vi "VI SysLog History.vi"() -> ()   [LabVIEW 2020, in "SysLog.lvlib"]
uses:
  SysLog.lvlib
  Stoerungen/Stoermelde Tabelle.ctl
  Visualisierungs Elemente/Button.ctl
  Visualisierungs Elemente/Auswahlfeld.ctl
  SysLogSort.ctl
  Passwortverwaltung/FGV Passwort Aktion.ctl
  <vilib>/Utility/miscctls.llb/LVRowAndColumnUnsignedTypeDef.ctl
  Allgemein/allgemeine Sub-VIs.lvlib
  Sprachverwaltung/Sprachverwaltung.lvlib
  Passwortverwaltung/Passwort.lvlib
  Stoerungen/Stoerungen.lvlib
panel:
  in  "SuchString":string caption="Suche"
  in  "interne":T1 items=["alle", "nur benutzerrelevante", "nur interne"]
  out "Fehler (out)":errorcluster caption="Fehlerkonstante"
  in  "cRIO History Laden":T2
  in  "PC History Laden":T2
  in  "Richtung":T1 items=["v", "^"]
  in  "Sortierung":T1 items=["Zeit", "Code", "Typ"]
  in  "Typ":T1 items=["*", "Err+Warn", "Err", "Warn", "OK"]
  in  "Ebene":T1 items=["PC+cRIO", "PC", "cRIO"]
  in  "refresh":T2 caption="quittieren"
  out "Tabelle":T3
  # "System Log History"
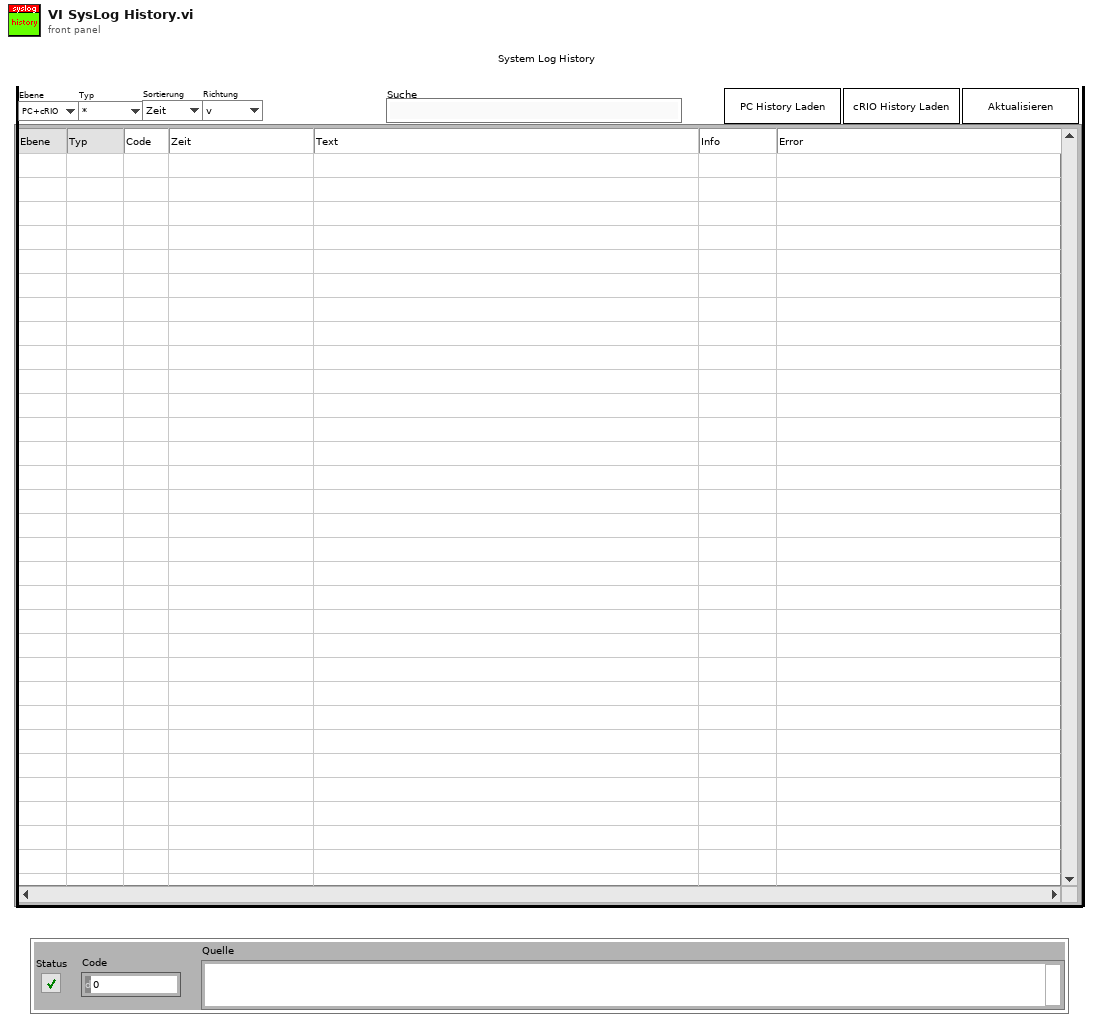
[diagram p1: front panel]
types:
  T1 = typedef "Auswahlfeld.ctl" = u16
  T2 = typedef "Button.ctl" = bool
  T3 = typedef "Stoerungen.lvlib/Stoermelde Tabelle.ctl" = string[][]
  T4 = typedef "Passwort.lvlib/FGV Passwort Aktion.ctl" = enum16{"prüfen", "setzen", "Initialisieren", "PW speichern", "lesen", "PW Änderung"}
  T5 = typedef "SysLog.lvlib/SysLogSort.ctl" = cluster{"interne":enum16{"alle", "nur benutzerrelevante", "nur interne"}, "Typ":enum16{"*", "Err+Warn", "Err", "Warn", "OK"}, "Sortierung":enum16{"Zeit", "Code", "Typ"}, "Richtung":enum16{"v", "^"}, "Filter":string}
  T6 = enum8{"Enabled", "Disabled", "Disabled and Grayed Out"}
  T7 = enum16{"alle", "nur benutzerrelevante", "nur interne"}
  T8 = typedef "LVRowAndColumnUnsignedTypeDef.ctl" = cluster{"Row":u32, "Column":u32}
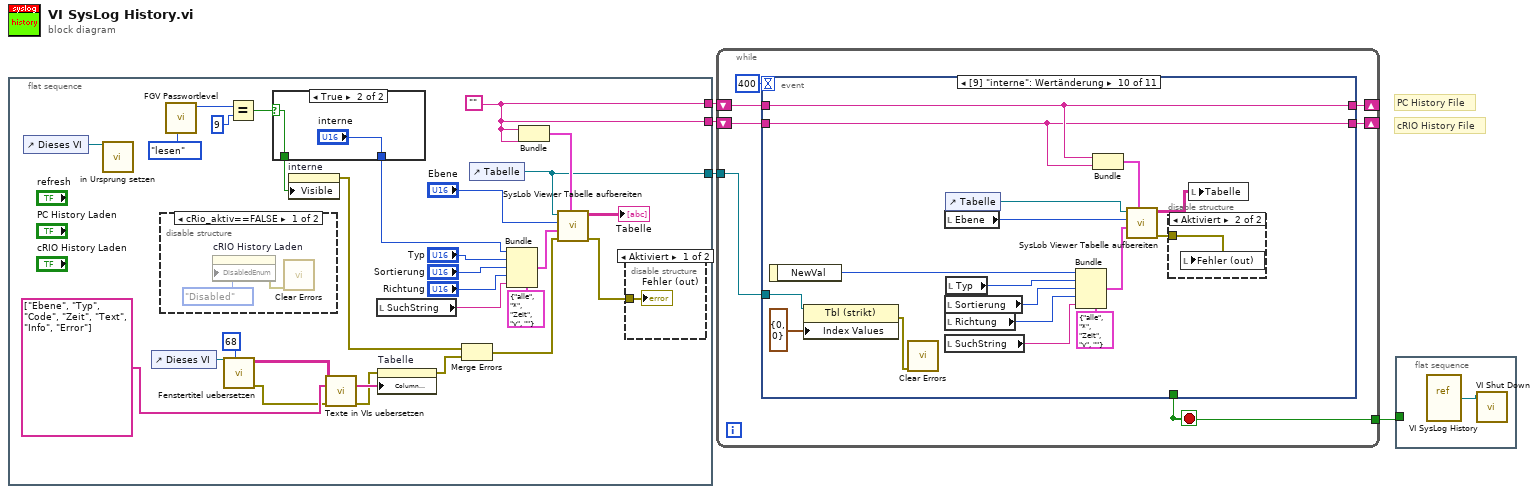
[diagram p0: block diagram]
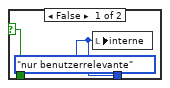
[diagram p2: hidden frame]
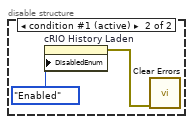
[diagram p3: hidden frame]
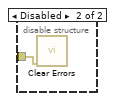
[diagram p4: hidden frame]
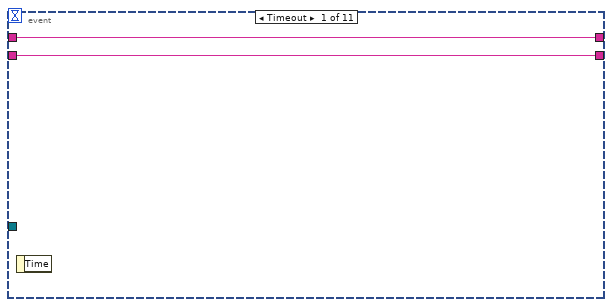
[diagram p5: hidden frame]
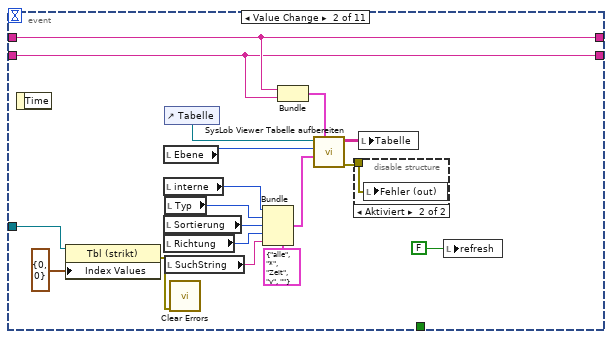
[diagram p6: hidden frame]
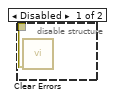
[diagram p7: hidden frame]
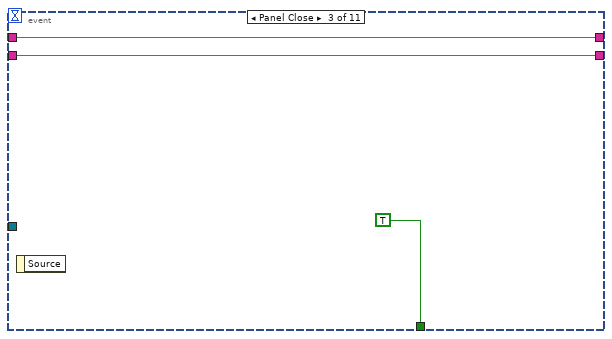
[diagram p8: hidden frame]
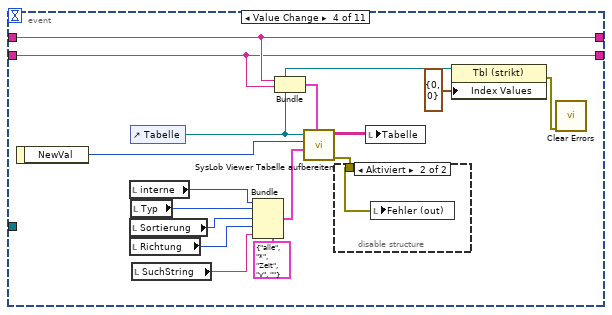
[diagram p9: hidden frame]
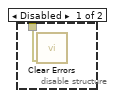
[diagram p10: hidden frame]
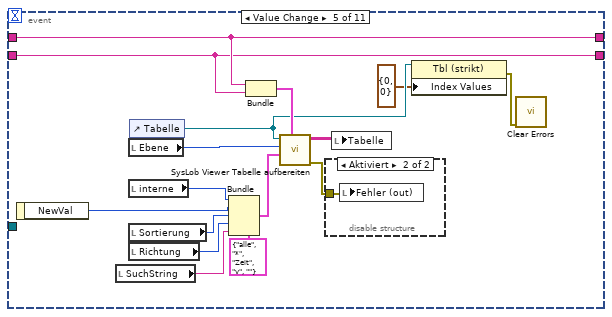
[diagram p11: hidden frame]
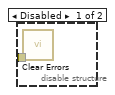
[diagram p12: hidden frame]
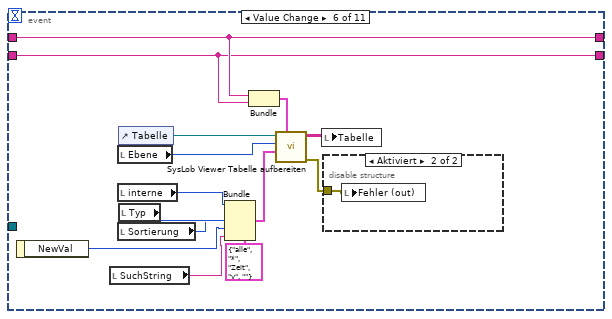
[diagram p13: hidden frame]
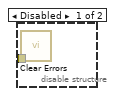
[diagram p14: hidden frame]
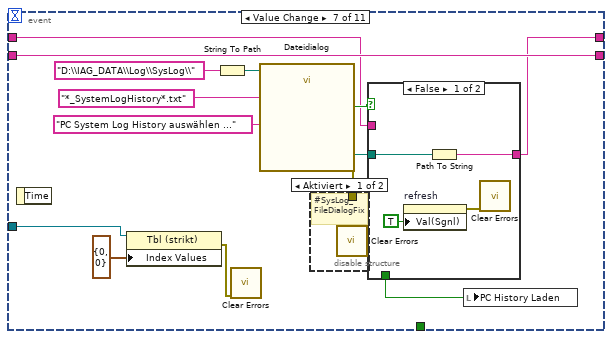
[diagram p15: hidden frame]
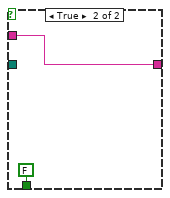
[diagram p17: hidden frame]
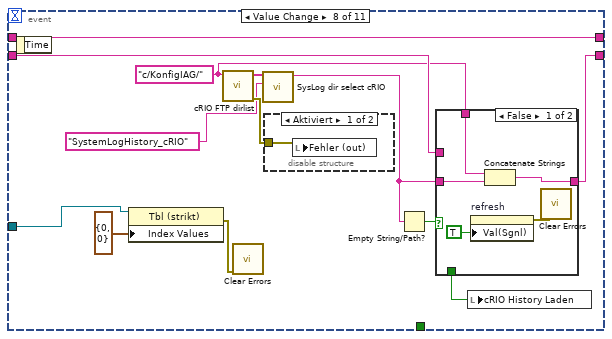
[diagram p18: hidden frame]
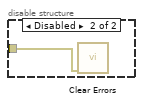
[diagram p19: hidden frame]
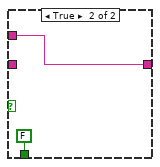
[diagram p20: hidden frame]
diagram:
  # "cRIO History File"
  # "PC History File"
  n1 = flat-sequence {
    tunnel: [w22] -> w3
    tunnel: [w22] -> w2
    tunnel: [w5] -> w1
    frame #0 {
      w22 = ""
      n2 = control-ref of="Dieses VI"() -> (w33:refnum<vi>)
      n3 = call "in Ursprung setzen.vi"("VI Referenz"=w33) -> ()  [unwired: 10 in, 1 out]
      n4 = control-ref of="Dieses VI"() -> (w16:refnum<vi>)
      n5 = disable-structure shown="cRio_aktiv==FALSE" {
        frame condition #0 {
          n6 = property on="cRIO History Laden" class="Bool. (strikt)"("DisabledEnum"=T6."Disabled" ("Deaktiviert")) -> (error out=w38:errorcluster)  [unwired: 2 in, 1 out]
          n7 = call <vilib>:"Clear Errors.vi"("error in (no error)"=w38) -> ()  [unwired: 5 in, 2 out]
        }
        frame condition #1 (active) {
          n8 = property on="cRIO History Laden" class="Bool. (strikt)"("DisabledEnum"=T6."Enabled" ("Deaktiviert")) -> (error out=w40:errorcluster)  [unwired: 2 in, 1 out]
          n9 = call <vilib>:"Clear Errors.vi"("error in (no error)"=w40) -> ()  [unwired: 5 in, 2 out]
        }
      }
      n10 = call "FGV Passwortlevel.vi"("FGV Passwort Aktion"=FGV_Passwort_Aktion."lesen") -> ("aktueller Level"=w19:i16)  [unwired: 3 in, 7 out]
      n11 = call "Fenstertitel uebersetzen.vi"("Index (Seite)"=68, "Dieses VI"=w16) -> ("error out"=w8:errorcluster, "Sprachliste"=w9:string[][])  [unwired: 6 in, 2 out]
      n12 = Equal?(x=w19, y=i16 9) -> (x = y?=w17:bool)
      n13 = case shown="True" w17 {
        selector: w17 -> [w35 w37]
        tunnel: [w35 w37] -> w11
        tunnel: [w34 "interne"] -> w10
        frame False {
          w34 = T7."nur benutzerrelevante" ("interne")
          n14 = local write "interne"(w34) -> ()
        }
        frame True {
        }
      }
      n15 = property on="interne" class="Ring (strikt)"("Visible"=w11) -> (error out=w12:errorcluster)  [unwired: 2 in, 1 out]
      n16 = call "Texte in VIs uebersetzen.vi"("Sprachliste"=w9, "String-Array zum Übersetzen"=string[] ["Ebene", "Typ", "Code", "Zeit", "Text", "Info", "Error"] ("Spaltentitel[]"), "error in (no error)"=w8) -> ("String-Array zum Übersetzen"=w31:string[], "error out"=w7:errorcluster)  [unwired: 8 in, 3 out]
      n17 = local read "SuchString"() -> (w6:string)
      n18 = property on="Tabelle" class="Tbl (strikt)"(error in=w7, "Column Headers[]"=w31) -> (error out=w14:errorcluster)  [unwired: 1 in, 1 out]
      n19 = Merge Errors(w12, w14) -> (w13:errorcluster)
      n20 = control-ref of="Tabelle"() -> (w5:refnum<vi>)
      n21 = Bundle(cluster=T5 {"interne"=enum."alle", "Typ"=enum."*", "Sortierung"=enum."Zeit", "Richtung"=enum."v", "Filter"=""} ("Cluster (in)"), "interne"=w10, "Typ"="Typ", "Sortierung"="Sortierung", "Richtung"="Richtung", "Filter"=w6) -> (w30:T5)
      n22 = Bundle(w22, w22) -> (w21:cluster{string, string})  [unwired: 1 in]
      n23 = call "SysLob Viewer Tabelle aufbereiten.vi"("Cluster PC cRIO History File"=w21, "Fehler (in)"=w13, "Cluster (in)"=w30, "Ebene"="Ebene", "Table (Eingang)"=w5) -> ("Fehler (out)"=w23:errorcluster, "Array-Typ (2D Dbl) out"=→"Tabelle":string[][])  [unwired: 5 in]
      n24 = disable-structure shown="Aktiviert" {
        disable-tunnel: w23 -> [w42 w43]
        frame Enabled {
          "Fehler (out)" <- w42
        }
        frame Disabled {
          n25 = call <vilib>:"Clear Errors.vi"("error in (no error)"=w43) -> ()  [unwired: 5 in, 2 out]
        }
      }
    }
  }
  n26 = while {
    tunnel: [w49] -> w4
    shift-right: [w47] -> _
    shift-left: w3 -> [w48]
    shift-right: [w45] -> _
    shift-left: w2 -> [w46]
    tunnel: w1 -> [w44]
    stop <- w49 stop-if-true
    n27 = event shown="[9] \"interne\": Wertänderung" {
      selector: _ -> [_ _ _ _ _ _ _ _ _ _ _]
      dyn-events: _ -> [_ _ _ _ _ _ _ _ _ _ _]
      timeout: 400 -> [_ _ _ _ _ _ _ _ _ _ _]
      tunnel: [_ _ TRUE _ _ _ _ _ _ _ _] -> w49
      tunnel: w48 -> [w52 w61 w74 w84 w101 w116 w134 w161 w175 w201 w219]
      tunnel: [w52 w61 w74 w84 w101 w116 w133 w161 w175 w201 w219] -> w47
      tunnel: w46 -> [w51 w60 w73 w83 w100 w115 w141 w160 w174 w200 w218]
      tunnel: [w51 w60 w73 w83 w100 w115 w141 w159 w174 w200 w218] -> w45
      tunnel: w44 -> [_ w53 _ _ _ _ w129 w149 _ w187 w206]
      event Timeout {
        n28 = event-data() -> ()  [unwired: 2 out]
      }
      event Value Change {
        n29 = event-data() -> ()  [unwired: 2 out]
        n30 = property class="Tbl (strikt)"(reference=w53, "Index Values"=T8 {"Row"=0, "Column"=0} ("Indexwerte")) -> (error out=w55:errorcluster)  [unwired: 1 in, 1 out]
        n31 = local read "Ebene"() -> (w67:T1)
        n32 = local read "interne"() -> (w57:T1)
        n33 = local read "Sortierung"() -> (w64:T1)
        n34 = local read "Richtung"() -> (w63:T1)
        n35 = control-ref of="Tabelle"() -> (w66:refnum<vi>)
        n36 = local read "Typ"() -> (w65:T1)
        n37 = local read "SuchString"() -> (w56:string)
        n38 = call <vilib>:"Clear Errors.vi"("error in (no error)"=w55) -> ()  [unwired: 5 in, 2 out]
        n39 = Bundle(cluster=T5 {"interne"=enum."alle", "Typ"=enum."*", "Sortierung"=enum."Zeit", "Richtung"=enum."v", "Filter"=""} ("Cluster (in)"), "interne"=w57, "Typ"=w65, "Sortierung"=w64, "Richtung"=w63, "Filter"=w56) -> (w70:T5)
        n40 = Bundle(w61, w60) -> (w59:cluster{string, string})  [unwired: 1 in]
        n41 = call "SysLob Viewer Tabelle aufbereiten.vi"("Cluster PC cRIO History File"=w59, "Cluster (in)"=w70, "Ebene"=w67, "Table (Eingang)"=w66) -> ("Fehler (out)"=w62:errorcluster, "Array-Typ (2D Dbl) out"=w68:string[][])  [unwired: 6 in]
        n42 = disable-structure shown="Aktiviert" {
          disable-tunnel: w62 -> [w71 w72]
          frame Disabled {
            n43 = call <vilib>:"Clear Errors.vi"("error in (no error)"=w71) -> ()  [unwired: 5 in, 2 out]
          }
          frame Enabled {
            n44 = local write "Fehler (out)"(w72) -> ()
          }
        }
        n45 = local write "Tabelle"(w68) -> ()
        n46 = local write "refresh"(FALSE) -> ()
      }
      event Panel Close {
        n47 = event-data() -> ()  [unwired: 2 out]
      }
      event Value Change {
        n48 = event-data() -> ("NewVal"=w89:T1)  [unwired: 1 out]
        n49 = local read "interne"() -> (w81:T1)
        n50 = local read "Sortierung"() -> (w87:T1)
        n51 = local read "Richtung"() -> (w86:T1)
        n52 = control-ref of="Tabelle"() -> (w77:refnum<vi>)
        n53 = local read "Typ"() -> (w88:T1)
        n54 = local read "SuchString"() -> (w80:string)
        n55 = Bundle(cluster=T5 {"interne"=enum."alle", "Typ"=enum."*", "Sortierung"=enum."Zeit", "Richtung"=enum."v", "Filter"=""} ("Cluster (in)"), "interne"=w81, "Typ"=w88, "Sortierung"=w87, "Richtung"=w86, "Filter"=w80) -> (w91:T5)
        n56 = Bundle(w84, w83) -> (w82:cluster{string, string})  [unwired: 1 in]
        n57 = call "SysLob Viewer Tabelle aufbereiten.vi"("Cluster PC cRIO History File"=w82, "Cluster (in)"=w91, "Ebene"=w89, "Table (Eingang)"=w77) -> ("Fehler (out)"=w85:errorcluster, "Array-Typ (2D Dbl) out"=w78:string[][])  [unwired: 6 in]
        n58 = disable-structure shown="Aktiviert" {
          disable-tunnel: w85 -> [w92 w93]
          frame Disabled {
            n59 = call <vilib>:"Clear Errors.vi"("error in (no error)"=w92) -> ()  [unwired: 5 in, 2 out]
          }
          frame Enabled {
            n60 = local write "Fehler (out)"(w93) -> ()
          }
        }
        n61 = local write "Tabelle"(w78) -> ()
        n62 = property class="Tbl (strikt)"(reference=w77, "Index Values"=T8 {"Row"=0, "Column"=0} ("Indexwerte")) -> (error out=w76:errorcluster)  [unwired: 1 in, 1 out]
        n63 = call <vilib>:"Clear Errors.vi"("error in (no error)"=w76) -> ()  [unwired: 5 in, 2 out]
      }
      event Value Change {
        n64 = event-data() -> ("NewVal"=w106:T1)  [unwired: 1 out]
        n65 = local read "SuchString"() -> (w97:string)
        n66 = local read "Ebene"() -> (w105:T1)
        n67 = local read "interne"() -> (w98:T1)
        n68 = local read "Sortierung"() -> (w104:T1)
        n69 = local read "Richtung"() -> (w103:T1)
        n70 = control-ref of="Tabelle"() -> (w95:refnum<vi>)
        n71 = Bundle(cluster=T5 {"interne"=enum."alle", "Typ"=enum."*", "Sortierung"=enum."Zeit", "Richtung"=enum."v", "Filter"=""} ("Cluster (in)"), "interne"=w98, "Typ"=w106, "Sortierung"=w104, "Richtung"=w103, "Filter"=w97) -> (w109:T5)
        n72 = Bundle(w101, w100) -> (w99:cluster{string, string})  [unwired: 1 in]
        n73 = call "SysLob Viewer Tabelle aufbereiten.vi"("Cluster PC cRIO History File"=w99, "Cluster (in)"=w109, "Ebene"=w105, "Table (Eingang)"=w95) -> ("Fehler (out)"=w102:errorcluster, "Array-Typ (2D Dbl) out"=w107:string[][])  [unwired: 6 in]
        n74 = disable-structure shown="Aktiviert" {
          disable-tunnel: w102 -> [w110 w111]
          frame Disabled {
            n75 = call <vilib>:"Clear Errors.vi"("error in (no error)"=w110) -> ()  [unwired: 5 in, 2 out]
          }
          frame Enabled {
            n76 = local write "Fehler (out)"(w111) -> ()
          }
        }
        n77 = local write "Tabelle"(w107) -> ()
        n78 = property class="Tbl (strikt)"(reference=w95, "Index Values"=T8 {"Row"=0, "Column"=0} ("Indexwerte")) -> (error out=w96:errorcluster)  [unwired: 1 in, 1 out]
        n79 = call <vilib>:"Clear Errors.vi"("error in (no error)"=w96) -> ()  [unwired: 5 in, 2 out]
      }
      event Value Change {
        n80 = event-data() -> ("NewVal"=w117:T1)  [unwired: 1 out]
        n81 = local read "SuchString"() -> (w112:string)
        n82 = local read "Ebene"() -> (w120:T1)
        n83 = local read "interne"() -> (w113:T1)
        n84 = local read "Sortierung"() -> (w118:T1)
        n85 = control-ref of="Tabelle"() -> (w121:refnum<vi>)
        n86 = local read "Typ"() -> (w119:T1)
        n87 = Bundle(cluster=T5 {"interne"=enum."alle", "Typ"=enum."*", "Sortierung"=enum."Zeit", "Richtung"=enum."v", "Filter"=""} ("Cluster (in)"), "interne"=w113, "Typ"=w119, "Sortierung"=w118, "Richtung"=w117, "Filter"=w112) -> (w125:T5)
        n88 = Bundle(w116, w115) -> (w114:cluster{string, string})  [unwired: 1 in]
        n89 = call "SysLob Viewer Tabelle aufbereiten.vi"("Cluster PC cRIO History File"=w114, "Cluster (in)"=w125, "Ebene"=w120, "Table (Eingang)"=w121) -> ("Fehler (out)"=w123:errorcluster, "Array-Typ (2D Dbl) out"=w122:string[][])  [unwired: 6 in]
        n90 = local write "Tabelle"(w122) -> ()
        n91 = disable-structure shown="Aktiviert" {
          disable-tunnel: w123 -> [w126 w127]
          frame Disabled {
            n92 = call <vilib>:"Clear Errors.vi"("error in (no error)"=w126) -> ()  [unwired: 5 in, 2 out]
          }
          frame Enabled {
            n93 = local write "Fehler (out)"(w127) -> ()
          }
        }
      }
      event Value Change {
        n94 = event-data() -> ()  [unwired: 2 out]
        n95 = property class="Tbl (strikt)"(reference=w129, "Index Values"=T8 {"Row"=0, "Column"=0} ("Indexwerte")) -> (error out=w131:errorcluster)  [unwired: 1 in, 1 out]
        n96 = String To Path(string="D:\\IAG_DATA\\Log\\SysLog\\") -> (path=w137:path)
        n97 = call <vilib>:"Clear Errors.vi"("error in (no error)"=w131) -> ()  [unwired: 5 in, 2 out]
        n98 = call "Dateidialog"("start path"=w137, "prompt"="PC System Log History auswählen ..." ("Eingabeaufforderung"), "pattern (all files)"="*_SystemLogHistory*.txt") -> ("selected path"=w135:path, "cancelled"=w136:bool, "error out"=w128:errorcluster)  [unwired: 9 in, 1 out]
        n99 = disable-structure shown="Aktiviert" {
          disable-tunnel: w128 -> [w142 _]
          frame Enabled {
            # "#SysLog_FileDialogFix"
            n100 = call <vilib>:"Clear Errors.vi"("error in (no error)"=w142) -> ()  [unwired: 5 in, 2 out]
          }
          frame Disabled {
          }
        }
        n101 = case shown="False" w136 {
          tunnel: w135 -> [w146 _]
          tunnel: [w145 w148] -> w133
          tunnel: w134 -> [_ w148]
          tunnel: [_ FALSE] -> w132
          frame False {
            n102 = property on="refresh" class="Bool. (strikt)"("Val(Sgnl)"=TRUE) -> (error out=w143:errorcluster)  [unwired: 2 in, 1 out]
            n103 = Path To String(path=w146) -> (string=w145:string)
            n104 = call <vilib>:"Clear Errors.vi"("error in (no error)"=w143) -> ()  [unwired: 5 in, 2 out]
          }
          frame True {
          }
        }
        n105 = local write "PC History Laden"(w132) -> ()
      }
      event Value Change {
        w152 = "c/KonfigIAG/" ("dir")
        n106 = event-data() -> ()  [unwired: 2 out]
        n107 = property class="Tbl (strikt)"(reference=w149, "Index Values"=T8 {"Row"=0, "Column"=0} ("Indexwerte")) -> (error out=w151:errorcluster)  [unwired: 1 in, 1 out]
        n108 = call "cRIO FTP dirlist.vi"("dir"=w152) -> ("Fehler (out)"=w156:errorcluster, "dir list"=w157:string[])  [unwired: 9 in]
        n109 = call <vilib>:"Clear Errors.vi"("error in (no error)"=w151) -> ()  [unwired: 5 in, 2 out]
        n110 = call "SysLog dir select cRIO.vi"("filter"="SystemLogHistory_cRIO" ("pattern (all files)"), "dir list"=w157) -> ("selected filename"=w155:string)  [unwired: 9 in]
        n111 = disable-structure shown="Aktiviert" {
          disable-tunnel: w156 -> [w162 w163]
          frame Enabled {
            n112 = local write "Fehler (out)"(w162) -> ()
          }
          frame Disabled {
            n113 = call <vilib>:"Clear Errors.vi"("error in (no error)"=w163) -> ()  [unwired: 5 in, 2 out]
          }
        }
        n114 = Empty String/Path?(string/path=w155) -> (empty?=w154:bool)
        n115 = case shown="False" w154 {
          tunnel: w155 -> [w168 _]
          tunnel: [w165 w170] -> w159
          tunnel: w160 -> [_ w170]
          tunnel: [_ FALSE] -> w158
          tunnel: w152 -> [w164 _]
          frame False {
            n116 = property on="refresh" class="Bool. (strikt)"("Val(Sgnl)"=TRUE) -> (error out=w166:errorcluster)  [unwired: 2 in, 1 out]
            n117 = Concatenate Strings(w164, w168) -> (w165:string)
            n118 = call <vilib>:"Clear Errors.vi"("error in (no error)"=w166) -> ()  [unwired: 5 in, 2 out]
          }
          frame True {
          }
        }
        n119 = local write "cRIO History Laden"(w158) -> ()
      }
      event Value Change {
        n120 = event-data() -> ("NewVal"=w178:T1)  [unwired: 1 out]
        n121 = local read "SuchString"() -> (w171:string)
        n122 = local read "Ebene"() -> (w180:T1)
        n123 = local read "interne"() -> (w172:T1)
        n124 = local read "Richtung"() -> (w177:T1)
        n125 = control-ref of="Tabelle"() -> (w182:refnum<vi>)
        n126 = local read "Typ"() -> (w179:T1)
        n127 = Bundle(cluster=T5 {"interne"=enum."alle", "Typ"=enum."*", "Sortierung"=enum."Zeit", "Richtung"=enum."v", "Filter"=""} ("Cluster (in)"), "interne"=w172, "Typ"=w179, "Sortierung"=w178, "Richtung"=w177, "Filter"=w171) -> (w183:T5)
        n128 = Bundle(w175, w174) -> (w173:cluster{string, string})  [unwired: 1 in]
        n129 = call "SysLob Viewer Tabelle aufbereiten.vi"("Cluster PC cRIO History File"=w173, "Cluster (in)"=w183, "Ebene"=w180, "Table (Eingang)"=w182) -> ("Fehler (out)"=w176:errorcluster, "Array-Typ (2D Dbl) out"=w181:string[][])  [unwired: 6 in]
        n130 = disable-structure shown="Aktiviert" {
          disable-tunnel: w176 -> [w185 w186]
          frame Disabled {
            n131 = call <vilib>:"Clear Errors.vi"("error in (no error)"=w185) -> ()  [unwired: 5 in, 2 out]
          }
          frame Enabled {
            n132 = local write "Fehler (out)"(w186) -> ()
          }
        }
        n133 = local write "Tabelle"(w181) -> ()
      }
      event Value Change {
        n134 = event-data() -> ("NewVal"=w199:T1)  [unwired: 1 out]
        n135 = property class="Tbl (strikt)"(reference=w187, "Index Values"=T8 {"Row"=0, "Column"=0} ("Indexwerte")) -> (error out=w189:errorcluster)  [unwired: 1 in, 1 out]
        n136 = call <vilib>:"Clear Errors.vi"("error in (no error)"=w189) -> ()  [unwired: 5 in, 2 out]
        n137 = local read "Ebene"() -> (w195:T1)
        n138 = local read "Sortierung"() -> (w193:T1)
        n139 = local read "Richtung"() -> (w192:T1)
        n140 = local read "SuchString"() -> (w190:string)
        n141 = control-ref of="Tabelle"() -> (w196:refnum<vi>)
        n142 = local read "Typ"() -> (w194:T1)
        n143 = Bundle(cluster=T5 {"interne"=enum."alle", "Typ"=enum."*", "Sortierung"=enum."Zeit", "Richtung"=enum."v", "Filter"=""} ("Cluster (in)"), "interne"=w199, "Typ"=w194, "Sortierung"=w193, "Richtung"=w192, "Filter"=w190) -> (w191:T5)
        n144 = Bundle(w201, w200) -> (w202:cluster{string, string})  [unwired: 1 in]
        n145 = call "SysLob Viewer Tabelle aufbereiten.vi"("Cluster PC cRIO History File"=w202, "Cluster (in)"=w191, "Ebene"=w195, "Table (Eingang)"=w196) -> ("Fehler (out)"=w198:errorcluster, "Array-Typ (2D Dbl) out"=w197:string[][])  [unwired: 6 in]
        n146 = disable-structure shown="Aktiviert" {
          disable-tunnel: w198 -> [w204 w205]
          frame Disabled {
            n147 = call <vilib>:"Clear Errors.vi"("error in (no error)"=w204) -> ()  [unwired: 5 in, 2 out]
          }
          frame Enabled {
            n148 = local write "Fehler (out)"(w205) -> ()
          }
        }
        n149 = local write "Tabelle"(w197) -> ()
      }
      event "SuchString": Value Change {
        n150 = event-data() -> ()  [unwired: 7 out]
        n151 = property class="Tbl (strikt)"(reference=w206, "Index Values"=T8 {"Row"=0, "Column"=0} ("Indexwerte")) -> (error out=w208:errorcluster)  [unwired: 1 in, 1 out]
        n152 = call <vilib>:"Clear Errors.vi"("error in (no error)"=w208) -> ()  [unwired: 5 in, 2 out]
        n153 = local read "Sortierung"() -> (w212:T1)
        n154 = local read "Ebene"() -> (w216:T1)
        n155 = control-ref of="Tabelle"() -> (w217:refnum<vi>)
        n156 = local read "Richtung"() -> (w211:T1)
        n157 = local read "interne"() -> (w214:T1)
        n158 = local read "Typ"() -> (w213:T1)
        n159 = Bundle(cluster=T5 {"interne"=enum."alle", "Typ"=enum."*", "Sortierung"=enum."Zeit", "Richtung"=enum."v", "Filter"=""} ("Cluster (in)"), "interne"=w214, "Typ"=w213, "Sortierung"=w212, "Richtung"=w211, "Filter"="SuchString") -> (w221:T5)
        n160 = Bundle(w219, w218) -> (w220:cluster{string, string})  [unwired: 1 in]
        n161 = call "SysLob Viewer Tabelle aufbereiten.vi"("Cluster PC cRIO History File"=w220, "Cluster (in)"=w221, "Ebene"=w216, "Table (Eingang)"=w217) -> ("Fehler (out)"=w215:errorcluster, "Array-Typ (2D Dbl) out"=w210:string[][])  [unwired: 6 in]
        n162 = disable-structure shown="Aktiviert" {
          disable-tunnel: w215 -> [w223 w224]
          frame Enabled {
            n163 = local write "Fehler (out)"(w223) -> ()
          }
          frame Disabled {
            n164 = call <vilib>:"Clear Errors.vi"("error in (no error)"=w224) -> ()  [unwired: 5 in, 2 out]
          }
        }
        n165 = local write "Tabelle"(w210) -> ()
      }
    }
  }
  n166 = flat-sequence {
    tunnel: w4 -> [_]
    frame #0 {
      n167 = vi-ref "VI SysLog History.vi"() -> (w225:refnum<vi>)
      n168 = call "VI Shut Down.vi"("VI Referenz"=w225) -> ()  [unwired: 11 in]
    }
  }
